vi "数据保存.vi"(9 "数值":dbl, 10 "数组":dbl[](array[numeric]), 11 "appended path":path) -> ()   [LabVIEW 2012]
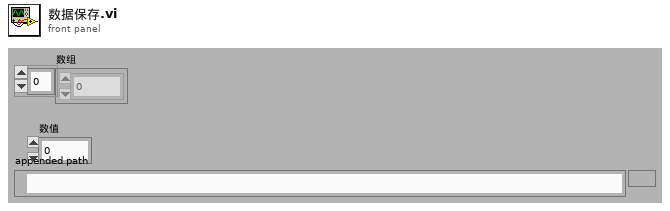
[diagram p1: front panel]
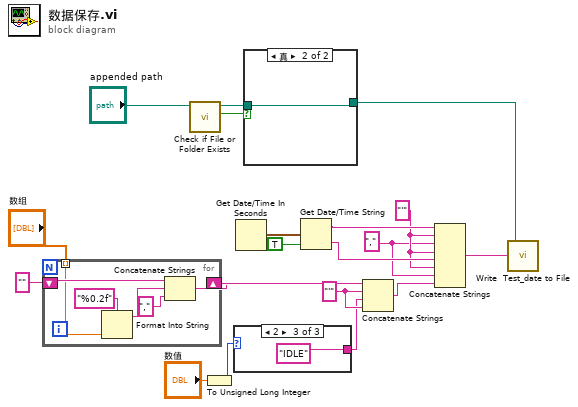
[diagram p0: block diagram]
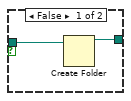
[diagram p2: hidden frame]
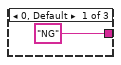
[diagram p3: hidden frame]
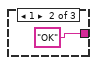
[diagram p4: hidden frame]
diagram:
  w15 = "'"
  w14 = ","
  w12 = "'" ("string")
  n1 = for {
    shift-right: [w24] -> w13
    shift-left: "" -> [w23]
    tunnel: "数组" -> [w20] mode=indexing
    n2 = Format Into String(format string="%0.2f", w20) -> (resulting string=w22:string)  [unwired: 2 in, 1 out]
    n3 = Concatenate Strings(w23, w22, "," ("string")) -> (w24:string)
  }
  n4 = call <vilib>:"Check if File or Folder Exists.vi"("path"="appended path") -> ("file or folder exists?"=w4:bool, "dup path"=w3:path)  [unwired: 8 in, 1 out]
  n5 = To Unsigned Long Integer(number="数值") -> (unsigned 32bit integer=w1:u32)
  n6 = case shown="2" w1 {
    tunnel: ["NG" "OK" "IDLE"] -> w11
    frame 0, Default {
    }
    frame 1 {
    }
    frame 2 {
    }
  }
  n7 = Get Date/Time In Seconds() -> (seconds since 1Jan1904=w9:timestamp)
  n8 = case shown="真" w4 {
    tunnel: w3 -> [w30 w31]
    tunnel: [w29 w31] -> w2
    frame False {
      n9 = Create Folder(path (use dialog)=w30) -> (created path=w29:path)  [unwired: 2 in, 2 out]
    }
    frame True {
    }
  }
  n10 = Get Date/Time String(seconds (now)=w9, want seconds? (F)=TRUE) -> (date string=w16:string, time string=w17:string)  [unwired: 1 in]
  n11 = Concatenate Strings(w13, w12, w11, w12) -> (w19:string)
  n12 = Concatenate Strings(w16, w15, w14, w15, w17, w15, w14, w19) -> (w18:string)
  n13 = call "Write  Test_date to File.vi"("String"=w18, "appended path"=w2) -> ()  [unwired: 3 in, 1 out]
